vi "api_mqttDisconnect.vi"(11 "error in (no error)":errorcluster) -> (15 "error out":errorcluster)   [LabVIEW 2020, in "mqtt.lvclass"]
uses:
  mqtt.lvclass
  mqttCmd/mqttCmdDisconnect/mqttCmdDisconnect.lvclass
  C:/Projects/Libraries/Gore SM 2020/mqtt-LabVIEW/src/class/mqtt/mqttCmd/mqttCmd.lvclass
panel:
  out "mqtt out":refnum<class "mqtt.lvclass">
  in  "mqtt in":refnum<class "mqtt.lvclass">
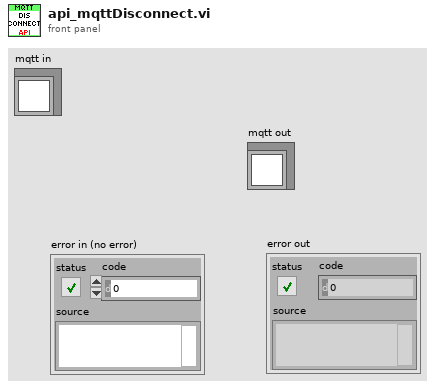
[diagram p1: front panel]
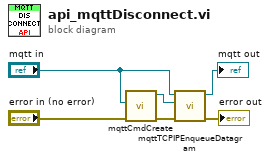
[diagram p0: block diagram]
diagram:
  n1 = call "mqttCmdCreate.vi"("error in (no error)"="error in (no error)", "mqtt instance"="mqtt in") -> ("error out"=w2:errorcluster, "mqttCmdDisconnect out"=w1:refnum<class "mqttCmdDisconnect.lvclass">)  [unwired: 8 in]
  n2 = call "mqttTCPIPEnqueueDatagram.vi"("error in (no error)"=w2, "mqttCmd"=w1, "mqtt in"="mqtt in") -> ("error out"=→"error out":errorcluster, "mqtt out"=→"mqtt out":refnum<class "mqtt.lvclass">)  [unwired: 7 in]
